vi "GrSimKickForce.vi"(10 "real kick":dbl) -> (2 "grsim kick":dbl)   [LabVIEW 2023]
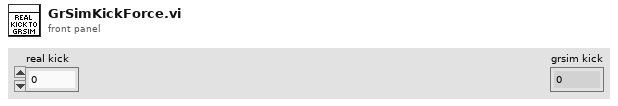
[diagram p1: front panel]
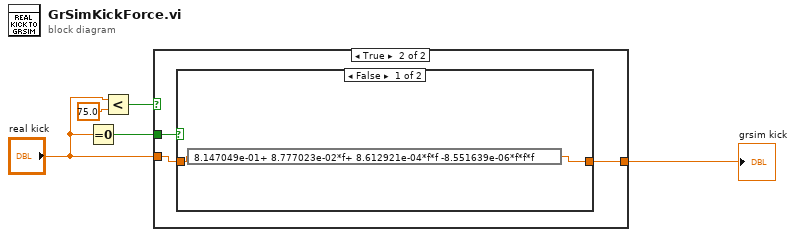
[diagram p0: block diagram]
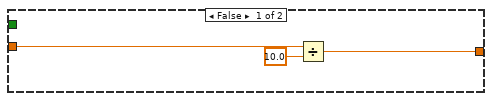
[diagram p2: hidden frame]
diagram:
  n1 = Equal To 0?(x="real kick") -> (x = 0?=w5:bool)
  n2 = Less?(x="real kick", y=75.0) -> (x < y?=w4:bool)
  n3 = case shown="True" w4 {
    tunnel: w5 -> [_ w11]
    tunnel: "real kick" -> [w8 w9]
    tunnel: [w7 w10] -> w1
    frame False {
      n4 = Divide(x=w8, y=10.0) -> (x/y=w7:dbl)
    }
    frame True {
      n5 = case shown="False" w11 {
        tunnel: [w13 w14] -> w10
        tunnel: w9 -> [w12 w14]
        frame False {
          n6 = expression code="8.147049e-01+ 8.777023e-02*f+ 8.612921e-04*f*f -8.551639e-06*f*f*f"(w12) -> (w13:dbl)
        }
        frame True {
        }
      }
    }
  }
  "grsim kick" <- w1
